vi "SmoothImage_V1.vi"(7 "Image IN":sgl[][](array[numeric]), 11 "Sigma (Radius)":dbl) -> (8 "Smoothed Image":sgl[][](array[numeric]))   [LabVIEW 2014]
uses:
  <vilib>/Analysis/2dsp.llb/2D Convolution (DBL).vi
  <vilib>/Analysis/NI_AALPro.lvlib
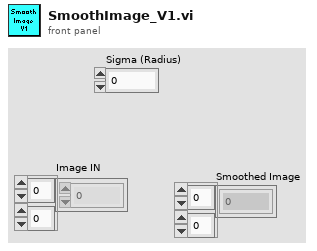
[diagram p1: front panel]
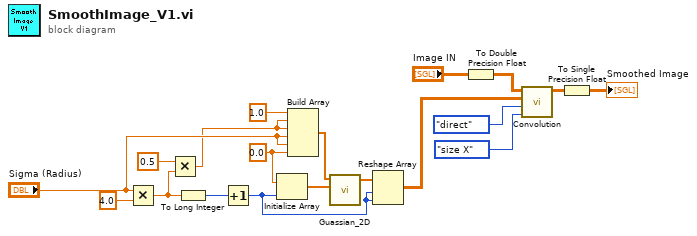
[diagram p0: block diagram]
diagram:
  w8 = 0.0 ("Numeric")
  n1 = Multiply(x="Sigma (Radius)", y=4.0) -> (x*y=w13:dbl)
  n2 = Multiply(x=0.5, y=w13) -> (x*y=w11:dbl)
  n3 = To Long Integer(number=w13) -> (32bit integer=w15:i32)
  n4 = Increment(x=w15) -> (x+1=w9:i32)
  n5 = Initialize Array(w8, w9) -> (w19:dbl[])
  n6 = Build Array(1.0 ("Numeric"), w11, w11, "Sigma (Radius)", "Sigma (Radius)", w8) -> (w10:dbl[])
  n7 = call "Guassian_2D.vi"("X"=w19, "a"=w10) -> ("f(X,a)"=w18:dbl[])  [unwired: 2 in, 2 out]
  n8 = Reshape Array(w18, w9, w9) -> (w5:dbl[][])
  n9 = To Double Precision Float(number="Image IN") -> (double precision float=w3:dbl[][])
  n10 = call-poly <vilib>:"Convolution.vi"("output size"=enum32{"full", "size X", "compact"}."size X", "algorithm"=enum32{"direct", "frequency domain"}."direct", "Y"=w5, "X"=w3) -> ("X * Y"=w2:dbl[][])  [unwired: 6 in, 1 out]
  n11 = To Single Precision Float(number=w2) -> (single precision float=→"Smoothed Image":sgl[][])
